vi "Global Mapper AJ.vi"(8 "Old Heading":dbl, 9 "Heading":dbl, 10 "Trail off/on":bool, 11 "GIC Input":T1={"     Use ?\nOff       On"=[FALSE, TRUE, FALSE, TRUE], "Mode:"=FALSE, "WP Data"="", "Hokuyo Port"="COM7", "Prop  Port"="COM6", "Compass Port"="", "GPS Port"="", "Num of WPs"=0, "WP Lats and Longs"={"WP Lats"=[], "WP Longs"=[]}, "Obst Lats and Longs"={"Obst Lats"=[], "Obst Longs"=[]}, "Parameters"=[], "GPS Data"=[], "Compass"=0.0, "LMS Vector"=[], "Vision Vector"=[], "Direction Cmd"=0.0, "Speed Cmd"=0.0, "WP Vector"=[], "WP Number"=0, "Extra"=0, "SW Map"=[], "Path Cluster"={"Path x node"=[], "Path y node"=[]}, "Sim Course"=[]} {"Obst Lats and Longs"."Obst Longs" format="%#_8g"; "Obst Lats and Longs"."Obst Lats" format="%#_8g"}) -> (0 "picture out":picture, 3 "Old Heading Out":dbl)   [LabVIEW 2014]
panel:
  in  "picture in":picture
  # "Global Mapper G"
  # "Inputs:"
  # "Output:"
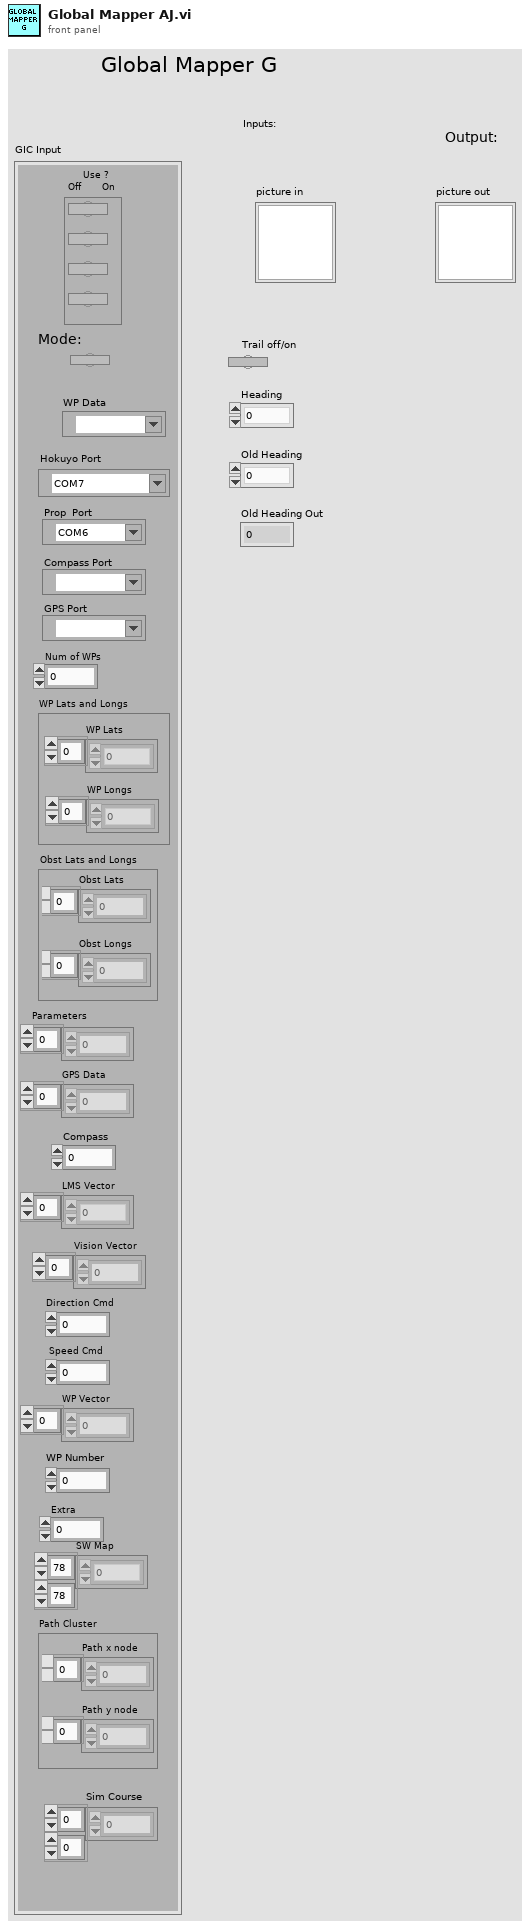
[diagram p1: front panel]
types:
  T1 = cluster{"     Use ?\nOff       On":bool[], "Mode:":bool, "WP Data":refnum<visa-resource-name>, "Hokuyo Port":refnum<visa-resource-name>, "Prop  Port":refnum<visa-resource-name>, "Compass Port":refnum<visa-resource-name>, "GPS Port":refnum<visa-resource-name>, "Num of WPs":i16, "WP Lats and Longs":cluster{"WP Lats":dbl[], "WP Longs":dbl[]}, "Obst Lats and Longs":cluster{"Obst Lats":dbl[], "Obst Longs":dbl[]}, "Parameters":dbl[], "GPS Data":dbl[], "Compass":dbl, "LMS Vector":dbl[], "Vision Vector":dbl[], "Direction Cmd":dbl, "Speed Cmd":dbl, "WP Vector":dbl[], "WP Number":i32, "Extra":i16, "SW Map":i32[][], "Path Cluster":cluster{"Path x node":dbl[], "Path y node":dbl[]}, "Sim Course":i8[][]}
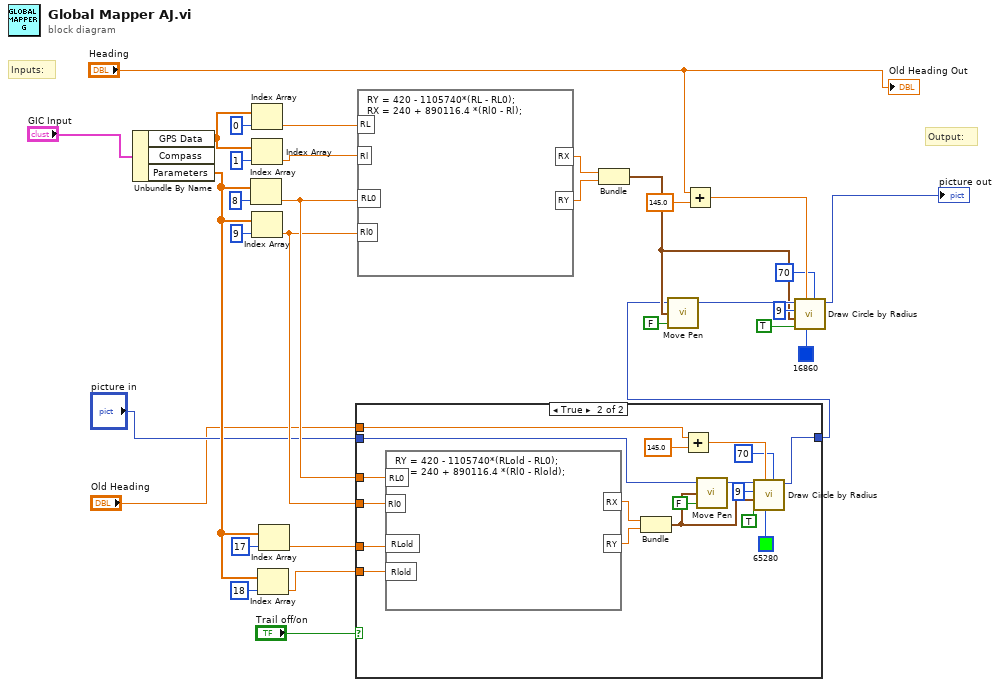
[diagram p0: block diagram]
diagram:
  # "Output:"
  # "Inputs:"
  n1 = Unbundle By Name("GIC Input") -> ("GPS Data"=w29:dbl[], "Parameters"=w14:dbl[])  [unwired: 1 out]
  n2 = Index Array(array=w14, index=8) -> (element=w12:dbl)
  n3 = Index Array(array=w29, index=0) -> (element=w31:dbl)
  n4 = Index Array(array=w29, index=1) -> (element=w27:dbl)
  n5 = Index Array(array=w14, index=9) -> (element=w11:dbl)
  n6 = Index Array(array=w14, index=18) -> (element=w9:dbl)
  n7 = Index Array(array=w14, index=17) -> (element=w10:dbl)
  n8 = case shown="True" "Trail off/on" {
    tunnel: w12 -> [_ w51]
    tunnel: w11 -> [_ w50]
    tunnel: w10 -> [_ w49]
    tunnel: w9 -> [_ w48]
    tunnel: [w33 w44] -> w7
    tunnel: "picture in" -> [w33 w38]
    tunnel: "Old Heading" -> [_ w37]
    frame False {
    }
    frame True {
      n9 = formula code="RY = 420 - 1105740*(RLold - RL0);\nRX = 240 + 890116.4 *(Rl0 - Rlold);"("RL0"=w51, "Rl0"=w50, "RLold"=w49, "Rlold"=w48) -> ("RX"=w47:dbl, "RY"=w46:dbl)
      n10 = Bundle("RX"=w47, "RY"=w46) -> (w43:cluster{"RX":dbl, "RY":dbl})  [unwired: 1 in]
      n11 = Add(x=w37, y=145.0) -> (x+y=w35:dbl)
      n12 = call <vilib>:"Move Pen.vi"("absolute coordinates?(T)"=FALSE, "new position"=w43, "picture"=w38) -> ("new picture"=w45:picture)  [unwired: 2 in]
      n13 = call <vilib>:"Draw Circle by Radius.vi"("arc size(360)"=i16 70, "color(black)"=u32 65280, "start angle(0)"=w35, "fill?(F)"=TRUE, "pixel center"=w43, "radius"=i16 9, "picture"=w45) -> ("new picture"=w44:picture)  [unwired: 4 in]
    }
  }
  n14 = formula code="RY = 420 - 1105740*(RL - RL0);\nRX = 240 + 890116.4 *(Rl0 - Rl);"("RL"=w31, "Rl"=w27, "RL0"=w12, "Rl0"=w11) -> ("RY"=w22:dbl, "RX"=w23:dbl)
  n15 = Bundle("RX"=w23, "RY"=w22) -> (w17:cluster{"RX":dbl, "RY":dbl})  [unwired: 1 in]
  n16 = call <vilib>:"Move Pen.vi"("absolute coordinates?(T)"=FALSE, "new position"=w17, "picture"=w7) -> ("new picture"=w24:picture)  [unwired: 2 in]
  n17 = Add(x="Heading", y=145.0) -> (x+y=w4:dbl)
  n18 = call <vilib>:"Draw Circle by Radius.vi"("arc size(360)"=i16 70, "color(black)"=u32 16860, "start angle(0)"=w4, "fill?(F)"=TRUE, "pixel center"=w17, "radius"=i16 9, "picture"=w24) -> ("new picture"=→"picture out":picture)  [unwired: 4 in]
  "Old Heading Out" <- "Heading"
